vi "Progress Indicator.vi"(11 "Main VI Ref":refnum<vi>) -> ()   [LabVIEW 2013, in "LVTM.lvlib"]
uses:
  LVTM.lvlib
panel:
  out "Progress":dbl(slide) caption="Adding VIs to tree" scale=0.0..4.0
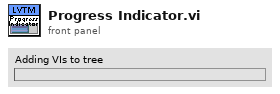
[diagram p1: front panel]
types:
  T1 = enum32{"Invalid", "Standard", "Closed", "Hidden", "Minimized", "Maximized"}
  T2 = typedef "LVRectTypeDef.ctl" = cluster{"Left":i16, "Top":i16, "Right":i16, "Bottom":i16}
  T3 = typedef "Status.ctl" = cluster{"Operation":string, "Total Interations":i32, "Current Iteration":i32, "Total Operations":i32, "Current Operation":i32}
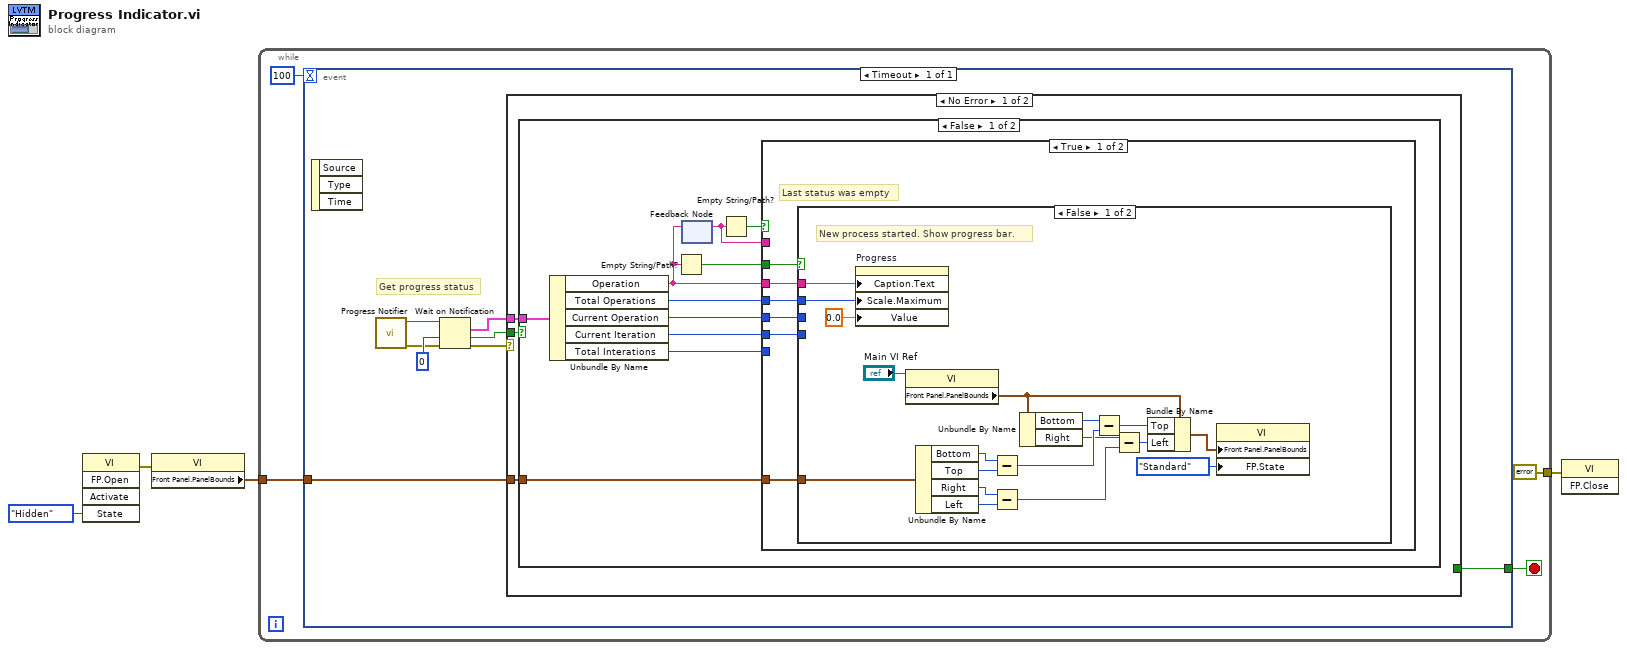
[diagram p0: block diagram]
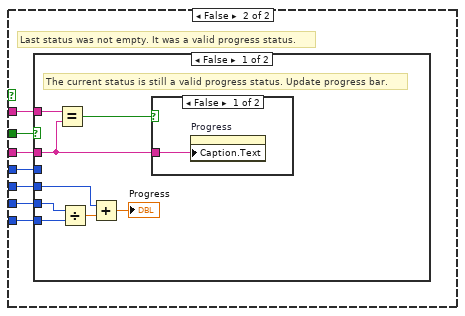
[diagram p3: hidden frame]
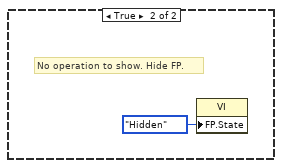
[diagram p5: hidden frame]
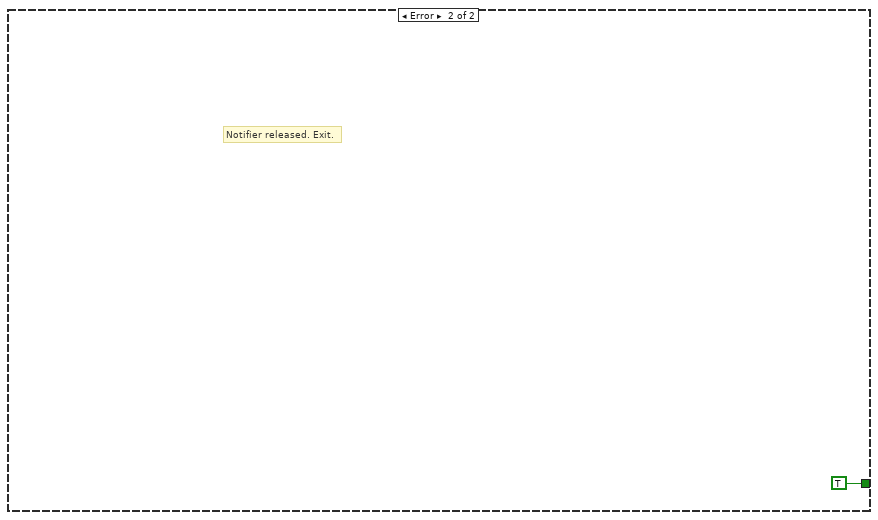
[diagram p7: hidden frame]
diagram:
  n1 = invoke class="VI" method="FP.Open"("State"=T1."Hidden") -> (error out=w3:errorcluster)  [unwired: 4 in, 4 out]
  n2 = property class="VI"(error in=w3) -> ("Front Panel.PanelBounds"=w2:T2)  [unwired: 1 in, 2 out]
  n3 = while {
    tunnel: w2 -> [w6]
    tunnel: [errorcluster {"status"=FALSE, "code"=0, "source"=""} ("error in (no error)")] -> w1
    stop <- w7 stop-if-true
    n4 = event shown="[0] Timeout" {
      selector: _ -> [_]
      dyn-events: _ -> [_]
      timeout: 100 -> [_]
      tunnel: [w10] -> w7
      tunnel: w6 -> [w9]
      event Timeout {
        # "Get progress status"
        n5 = event-data() -> ()  [unwired: 1 in, 3 out]
        n6 = call "Progress Notifier.vi"() -> ("error out"=w14:errorcluster, "notifier out"=w16:refnum<notifier>)  [unwired: 10 in]
        n7 = Wait on Notification(notifier=w16, timeout in ms (-1)=0, error in (no error)=w14) -> (notification=w12:T3, timed out?=w13:bool, error out=w11:errorcluster)  [unwired: 1 in, 1 out]
        n8 = case shown="No Error" w11 {
          tunnel: w13 -> [w19 _]
          tunnel: w12 -> [w18 _]
          tunnel: [_ TRUE] -> w10
          tunnel: w9 -> [w17 _]
          frame No Error {
            n9 = case shown="False" w19 {
              tunnel: w18 -> [w26 _]
              tunnel: w17 -> [w20 _]
              frame False {
                n10 = Unbundle By Name(w26) -> ("Operation"=w24:string, "Total Operations"=w29:i32, "Current Operation"=w28:i32, "Current Iteration"=w27:i32, "Total Interations"=w22:i32)
                n11 = Empty String/Path?(string/path=w24) -> (empty?=w23:bool)
                n12 = feedback-in #1(w24) -> ()
                n13 = feedback #1() -> (w21:string)  [unwired: 1 in]
                n14 = Empty String/Path?(string/path=w21) -> (empty?=w25:bool)
                n15 = case shown="True" w25 {
                  tunnel: w29 -> [w31 w56]
                  tunnel: w28 -> [w32 w60]
                  tunnel: w27 -> [w33 w59]
                  tunnel: w24 -> [w34 w58]
                  tunnel: w23 -> [w35 w57]
                  tunnel: w22 -> [_ w55]
                  tunnel: w21 -> [_ w54]
                  tunnel: w20 -> [w30 _]
                  frame True {
                    # "Last status was empty"
                    n16 = case shown="False" w35 {
                      tunnel: w34 -> [w53 _]
                      tunnel: w33 -> [_ _]
                      tunnel: w32 -> [_ _]
                      tunnel: w31 -> [w51 _]
                      tunnel: w30 -> [w40 _]
                      frame False {
                        # "New process started. Show progress bar."
                        n17 = property on="Progress" class="Slide (strict)"("Caption.Text"=w53, "Scale.Maximum"=w51, "Value"=0.0 ("Progress")) -> ()  [unwired: 2 in, 2 out]
                        n18 = property class="VI"(reference="Main VI Ref") -> ("Front Panel.PanelBounds"=w44:T2)  [unwired: 1 in, 2 out]
                        n19 = Unbundle By Name(w40) -> ("Bottom"=w47:i16, "Top"=w48:i16, "Right"=w45:i16, "Left"=w46:i16)
                        n20 = Subtract(x=w47, y=w48) -> (x-y=w42:i16)
                        n21 = Subtract(x=w45, y=w46) -> (x-y=w38:i16)
                        n22 = Unbundle By Name(w44) -> ("Bottom"=w43:i16, "Right"=w39:i16)
                        n23 = Subtract(x=w43, y=w42) -> (x-y=w41:i16)
                        n24 = Subtract(x=w39, y=w38) -> (x-y=w37:i16)
                        n25 = Bundle By Name(cluster=w44, "Top"=w41, "Left"=w37) -> (w36:T2)
                        n26 = property class="VI"("Front Panel.PanelBounds"=w36, "FP.State"=T1."Standard" ("Front Panel Window:State")) -> ()  [unwired: 2 in, 2 out]
                      }
                      frame True {
                        # "New status is empty. Do nothing."
                      }
                    }
                  }
                  frame False {
                    # "Last status was not empty. It was a valid progress status."
                    n27 = case shown="False" w57 {
                      tunnel: w58 -> [w62 _]
                      tunnel: w60 -> [w66 _]
                      tunnel: w59 -> [w68 _]
                      tunnel: w56 -> [_ _]
                      tunnel: w55 -> [w67 _]
                      tunnel: w54 -> [w63 _]
                      frame False {
                        # "The current status is still a valid progress status. Update progress bar."
                        n28 = Equal?(x=w63, y=w62) -> (x = y?=w61:bool)
                        n29 = Divide(x=w68, y=w67) -> (x/y=w65:dbl)
                        n30 = Add(x=w66, y=w65) -> (x+y=→"Progress":dbl)
                        n31 = case shown="False" w61 {
                          tunnel: w62 -> [w69 _]
                          frame False {
                            n32 = property on="Progress" class="Slide (strict)"("Caption.Text"=w69) -> ()  [unwired: 2 in, 2 out]
                          }
                          frame True {
                          }
                        }
                      }
                      frame True {
                        # "No operation to show. Hide FP."
                        n33 = property class="VI"("FP.State"=T1."Hidden" ("Front Panel Window:State")) -> ()  [unwired: 2 in, 2 out]
                      }
                    }
                  }
                }
              }
              frame True {
                # "timed out, no new status"
              }
            }
          }
          frame Error {
            # "Notifier released. Exit."
          }
        }
      }
    }
  }
  n34 = invoke class="VI" method="FP.Close"(error in=w1) -> ()  [unwired: 2 in, 3 out]
